vi "tcsWEP_logEvent_imageReady.vi"(8 "error in (no error)":errorcluster, 11 "logevent_imageReady_Ctl":T1) -> (0 "error out":errorcluster, 2 "function return":i32, 3 "logevent_imageReady_Ctl out":T1)   [LabVIEW 2016, in "SALLV_tcsWEP.lvlib"]
doc: "int tcsWEP_shm_logEvent_imageReadyLV(tcsWEP_logevent_imageReadyLV *logevent_imageReady_Ctl );"
uses:
  SALLV_tcsWEP.lvlib
  DataTypes/logevent_imageReady.ctl
  SALLV_tcsWEP.so
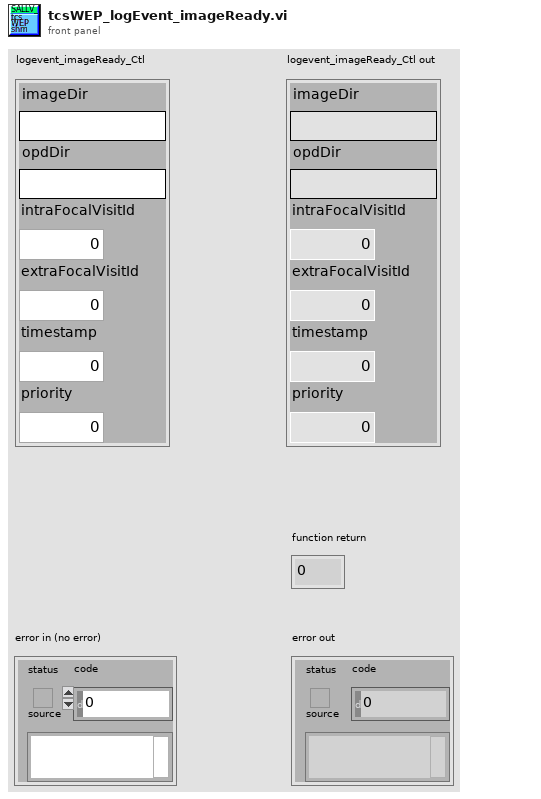
[diagram p1: front panel]
types:
  T1 = typedef "SALLV_tcsWEP.lvlib/logevent_imageReady.ctl" = cluster{"imageDir":string, "opdDir":string, "intraFocalVisitId":i32, "extraFocalVisitId":i32, "timestamp":dbl, "priority":i32}
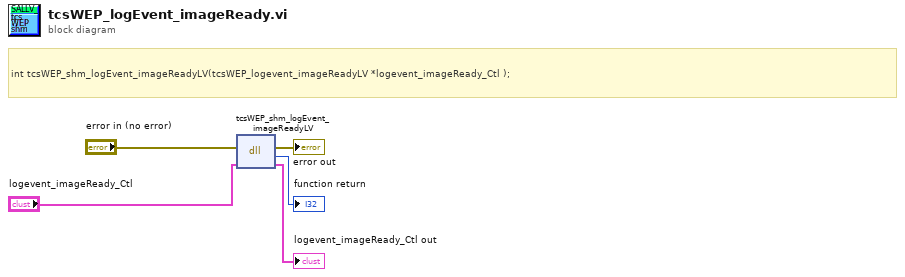
[diagram p0: block diagram]
diagram:
  # "int tcsWEP_shm_logEvent_imageReadyLV(tcsWEP_logevent_imageReadyLV *logevent_imageReady_Ctl );"
  n1 = dll-call lib="home/ttsai/Documents/salAPI/SALLV_tcsWEP.*" fn="tcsWEP_shm_logEvent_imageReadyLV"(error in="error in (no error)", "logevent_imageReady_Ctl"="logevent_imageReady_Ctl") -> (error out=→"error out":errorcluster, →"function return":i32, "logevent_imageReady_Ctl"=→"logevent_imageReady_Ctl out":T1)  [unwired: 2 in, 1 out]
